vi "LS4 SetDimensions_SD.vi"(1 "AD":i32, 2 "ZD":i32, 3 "YD":i32, 4 "XD":i32) -> (0 "Command executed":bool)   [LabVIEW 2015]
doc: "Selects the dimension of the position values (separate for each axis).\n\n0 = MicroSteps\n1 = um\n2 = mm"
uses:
  DLL/LStep4.dll
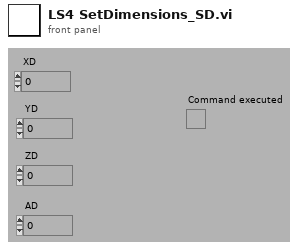
[diagram p1: front panel]
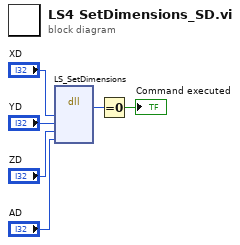
[diagram p0: block diagram]
diagram:
  n1 = dll-call lib="G:/SD/TRANCON-2015/DLL/LStep4.dll" fn="LS_SetDimensions"("XD"="XD", "YD"="YD", "ZD"="ZD", "AD"="AD") -> ("type de retour"=w2:i32)  [unwired: 7 in, 2 out]
  n2 = Equal To 0?(x=w2) -> (x = 0?=→"Command executed":bool)
